vi "AlliGator Reject Source Image ROIs based on Characteristics.vi"(8 "error in (no error)":errorcluster, 10 "ROI Mask Refnum":T1, 11 "Source Image Refnum":T1) -> (0 "error out":errorcluster, 1 "ROI Characteristics String":string)   [LabVIEW 2021, in "AlliGator ROIs.lvlib"]
doc: "Computes ROI characteristics and compare them to the conditions defined by the user in a dialog box.\n\nKeeps only the ROIs that meet those conditions."
uses:
  AlliGator ROIs.lvlib
  <vilib>/vision/Image Controls.llb/IMAQ Image.ctl
  Globals, Variables, Constants/AlliGator Variables List.ctl
  Image/Named ROI Description.ctl
  AlliGator ROI Manager Actions.ctl
  AlliGator Source Image ROI Storage [SGL] v3.vi
  Globals, Variables, Constants/AlliGator Globals, Variables & Constants.lvlib
  Image/Image.lvlib
  Source Image/AlliGator Source Image.lvlib
  Strings/Strings.lvlib
panel:
  # "see the AlliGator License on the block diagram (Ctrl+E or Window:Show Block Diagram)"
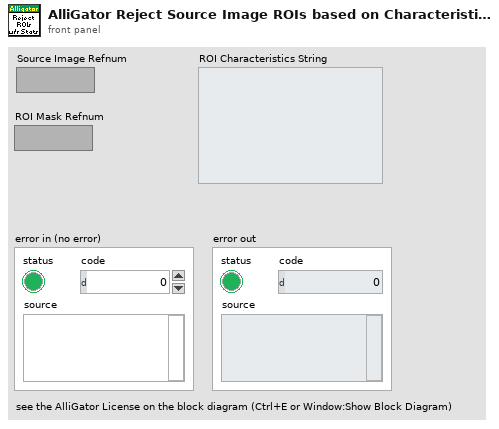
[diagram p1: front panel]
types:
  T1 = typedef "IMAQ Image.ctl" = refnum<image>
  T2 = typedef "Image.lvlib/Named ROI Description.ctl" = cluster{"ROI Descriptor":T3, "ROI Name":string, "Overlay Color":u32}
  T3 = typedef "ROI Descriptor" = cluster{"Global Rectangle":i32[], "Contours":cluster{"ID":enum32{"External", "Internal"}, "Type":u32, "Coordinates":i32[]}[]}
  T4 = typedef "AlliGator Globals, Variables & Constants.lvlib/AlliGator Variables List.ctl" = enum16{"---- GUI ----", "GUI:Initialization Status", "GUI:State Indicators Refnum", "GUI:Original AlliGator Menu Items", "GUI:Current Action Loop State", "GUI:Script in progress", "GUI:Playback", "GUI:Loop Playback", "GUI:Search ROI Used", "GUI:Search ROI", "Decay Graph Max Legend Size", "Intensity Graph Max Legend Size", "Decay Statistics Graph Max Legend Size", "Phasor Graph Max Legend Size", "Phasor Ratio Graph Max Legend Size", "Lifetime Graph Max Legend Size", "---- Files ----", "Files:Export Dataset Frames as Individual Files", "Files:Show Batch Export Help Balloons", "Files:Frames in Dataset", "Files:ptu File Frame Start Indices", "Files:Current Frame in Dataset", "Files:Current Frame Timestamp", "Files:Dataset Loaded", "Files:Dataset Metadata", "Files:Dataset Channel", "Files:Dataset Data Description", "Files:Background Dataset Metadata", "Files:Background Dataset Channel", "Files:Background Dataset Data Description", "Files:Background File Subtraction", "Files:Background File Path", "Files:Background File Pile-up Correction", "Files:Background File Pixel Well Capacity", "Files:Background File Scaling Factor", "Files:Current Dataset Load Settings", "Files:Dataset Path", "Files:ICCD-specific Information", "Files:Macrotime Gate Separation", "------ Python Plugins ------", "Python Plugins:Information", "Python Plugins:Python Session", "Python Plugins:Valid Python Session?", "---- Source Image ----", "Source Image:ROIs", "Source Image:Current ROI", "Source Image:ROI Event Refnum", "X_Source Image Display Range", "X_Source Image Palette Information", "X_Type of Displayed Image", "X_Time Gate Slider", "Source Image:Palette List", "Source Image:Scale", "Source Image:ROI Overlay Color", "Source Image:Overlay to Erase", "Source Image:Is Displayed Image Accumulated", "Source Image:White Light Image Modified", "Source Image:Mask Image Modified", "---- Image Profile Window ----", "Image Profile:Window Event Refnum", "Image Profile:IntensityType", "Image Profile:Intensity Average Type", "Image Profile:Intensity-weighted SDV", "Image Profile:Box Profile Type", "Image Profile:Window Open", "Image Profile:Plotted Fit Parameter", "------ Phasor Graph -------", "Phasor Graph:Show Line", "---- Phasor Plot ---", "Phasor Plot:Parameters Changed", "Phasor Plot:FLI Dataset Modified since last Calculation", "Phasor Harmonics Data", "Selected Phasor Harmonics", "Phasor Harmonic Manager Event Refnum", "Phasor Plot:ROIs", "Phasor Plot:Current ROI", "Phasor Plot:ROI Event Refnum", "Phasor Plot:Image Reference Points", "Phasor Plot:Computed", "Phasor Plot:Palette Information", "Phasor Plot:Palette List", "Phasor Plot:Phasor Ratio Palette Information", "Phasor Plot:Phasor Ratio Palette List", "Phasor Plot:Image Scale", "Phasor Plot:Image Overlay to Erase", "Phasor Plot:Image Elements to Update", "Phasor Plot:Current Calculation Parameters", "Phasor Plot:Current Calibration Options", "Phasor Plot:Reset Cumulated Phasor Plot", "Phasor Plot:Reference 1", "Phasor Plot:Lifetime Reference 1", "Phasor Plot:Reference 1 Frequency", "Phasor Plot:Reference 2", "Phasor Plot:Lifetime Reference 2", "Phasor Plot:Reference 2 Frequency", "---- Decay Analysis ----", "Number of Selected Decays to Fit", "LS Fit Results", "LAR Fit Results", "BS Fit Results", "Last Decay Max - Min", "Best Fit Parameters", "Best Fit Parameter Names", "Actual Size X", "Actual Size Y", "Binning X", "Binning Y", "Actual # Gates", "Dataset Number", "Gates to...", "Gates Skipped", "Gates to keep", "Gate Step", "Gate Separation", "Reversed Gates", "Pile-up Correction", "Pixel Well Capacity", "Background Subtracted", "Background Subtraction Method", "Background Definition Range", "Background File (deprecated)", "Number of Dataset Accumulated", "Array of Accumulated Dataset Paths", "Do Averaged Datasets", "Destination File Path", "Process Plot Target", "Use 1/D as Phasor Frequency", "---- Decay Fit Parameter Map -----", "Decay Fit Parameter Map:Palette Information", "Decay Fit Parameter Map:Palette List", "---- Parameter Map ----", "Parameter Map:Palette Information", "Parameter Map:Palette List", "------- Local Decay Window ---------", "Local Decay Graph Window:Event Refnum", "Local Decay Graph Window:Use normalized IRF for convolution", "----- Miscellaneous ----", "Misc:Skippable Dialog Windows Status"}
  T5 = typedef "AlliGator ROIs.lvlib/AlliGator ROI Manager Actions.ctl" = enum16{"Undefined", "Delete Current ROI", "Delete All Unselected ROIs", "Delete Multiple ROIs", "Delete All ROIs", "Swap ROIs", "Insert ROI", "Update Current ROI Descriptor", "Rename Current ROI", "Store New ROI", "Store Multiple ROIs", "Select Next ROI", "Select Previous ROI", "Find Selected ROI", "Show All ROIs", "Update ROI Manager Window", "Merge All ROIs", "Unmerge ROI", "Set Selected ROI by ID"}
  T6 = typedef "Image.lvlib/Image ROI Statistics.ctl" = cluster{"Area (pixels)":dbl, "% of Image":dbl, "Total Intensity":dbl, "Mean Intensity":dbl, "Median Intensity":dbl, "Mode Intensity":dbl, "Intensity Standard Deviation":dbl, "Min Intensity":dbl, "Max Intensity":dbl, "Mean SNR":dbl, "Median SNR":dbl, "Mode SNR":dbl, "SNR Standard Deviation":dbl, "Max SNR":dbl, "Min SNR":dbl, "# Rejected Pixels (NaN, Inf)":dbl, "# Negative Pixels":dbl, "Long Axis Length":dbl, "Short Axis Length":dbl, "Aspect Ratio":dbl}
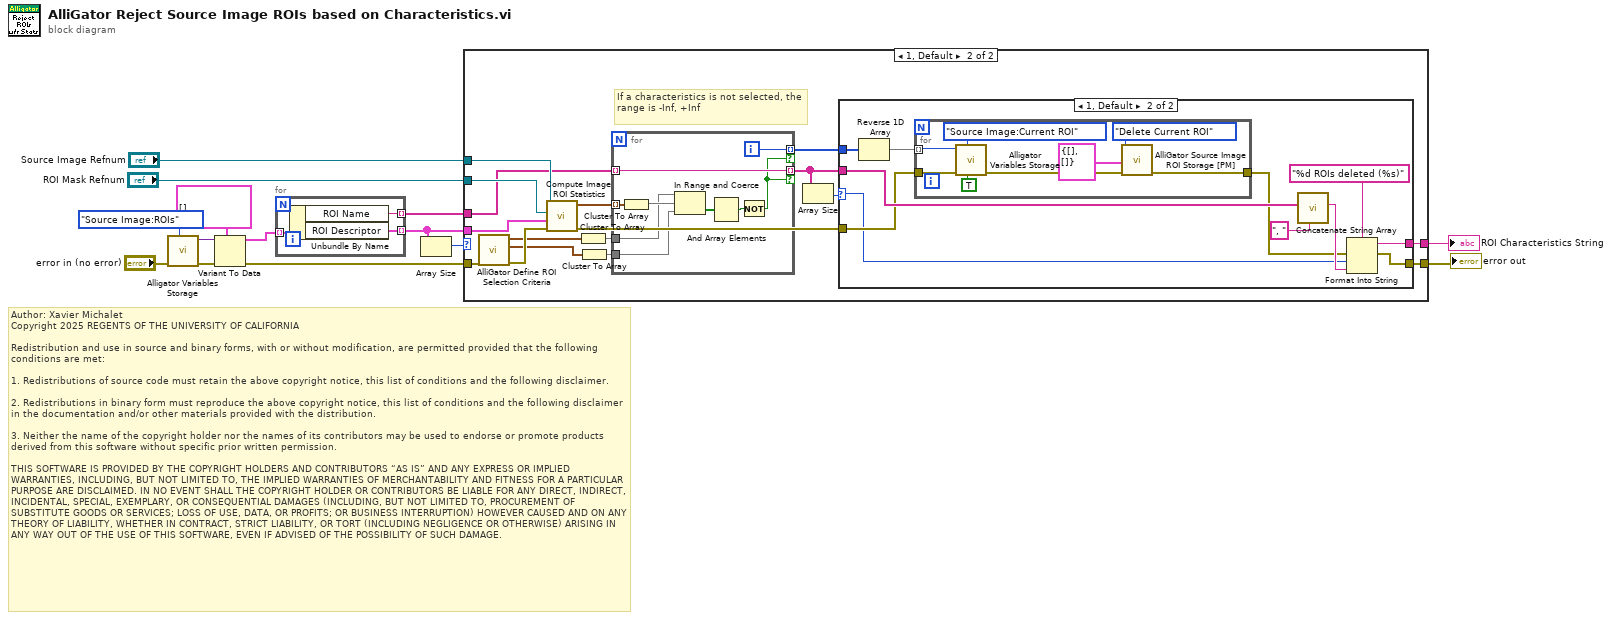
[diagram p0: block diagram]
diagram:
  # "Author: Xavier Michalet\nCopyright 2025 REGENTS OF THE UNIVERSITY OF CALIFORNIA\n\nRedistribution and use in source and binary forms, with or without modification, are permitted provided that the following conditions are met:\n\n1. Redistributions of source code must retain the above copyright notice, this list of conditions and the following disclaimer.\n\n2. Redistributions in binary form must reproduce the above copyright notice, this list of conditions and the following disclaimer in the documentation and/or other materials provided with the distribution.\n\n3. Neither the name of the copyright holder nor the names of its contributors may be used to endorse or promote products derived from this software without specific prior written permission.\n\nTHIS SOFTWARE IS PROVIDED BY THE COPYRIGHT HOLDERS AND CONTRIBUTORS “AS IS” AND ANY EXPRESS OR IMPLIED WARRANTIES, INCLUDING, BUT NOT LIMITED TO, THE IMPLIED WARRANTIES OF MERCHANTABILITY AND FITNESS FOR A PARTICULAR PURPOSE ARE DISCLAIMED. IN NO EVENT SHALL THE COPYRIGHT HOLDER OR CONTRIBUTORS BE LIABLE FOR ANY DIRECT, INDIRECT, INCIDENTAL, SPECIAL, EXEMPLARY, OR CONSEQUENTIAL DAMAGES (INCLUDING, BUT NOT LIMITED TO, PROCUREMENT OF SUBSTITUTE GOODS OR SERVICES; LOSS OF USE, DATA, OR PROFITS; OR BUSINESS INTERRUPTION) HOWEVER CAUSED AND ON ANY THEORY OF LIABILITY, WHETHER IN CONTRACT, STRICT LIABILITY, OR TORT (INCLUDING NEGLIGENCE OR OTHERWISE) ARISING IN ANY WAY OUT OF THE USE OF THIS SOFTWARE, EVEN IF ADVISED OF THE POSSIBILITY OF SUCH DAMAGE."
  n1 = call "Alligator Variables Storage.vi"("AlliGator Variable"=AlliGator_Variables_List."Source Image:ROIs" ("Alligator Variable"), "Error In"="error in (no error)") -> ("Error Out"=w10:errorcluster, "Data out"=w9:variant)  [unwired: 7 in, 1 out]
  n2 = Variant To Data(error in=w10, type=T2[] [] ("Stored ROIs in"), Variant=w9) -> (data=w12:T2[], error out=w5:errorcluster)
  n3 = for {
    tunnel: w12 -> [w17] mode=indexing
    tunnel: [w16] -> w3 mode=indexing
    tunnel: [w15] -> w1 mode=indexing
    n4 = Unbundle By Name(w17) -> ("ROI Name"=w15:string, "ROI Descriptor"=w16:T3)
  }
  n5 = Array Size(array=w3) -> (size(s)=w2:i32)
  n6 = case shown="1, Default" w2 {
    tunnel: "ROI Mask Refnum" -> [_ w35]
    tunnel: "Source Image Refnum" -> [_ w34]
    tunnel: [w18 w32] -> w7
    tunnel: [_ w31] -> w6
    tunnel: w5 -> [w18 w30]
    tunnel: w3 -> [_ w28]
    tunnel: w1 -> [_ w24]
    frame 0 {
      # "no ROIs"
    }
    frame 1, Default {
      # "If a characteristics is not selected, the range is -Inf, +Inf"
      n7 = call "AlliGator Define ROI Selection Criteria.vi"("Error In"=w30) -> ("Error Out"=w29:errorcluster, "ROI Characteristics Min out"=w19:T6, "ROI Characteristics Max out"=w27:T6)  [unwired: 7 in, 1 out]
      n8 = call "Compute Image ROI Statistics.vi"("error in (no error)"=w29, "ROIs"=w28, "ROI Mask Refnum"=w35, "Image Refnum"=w34) -> ("error out"=w23:errorcluster, "ROI Characteristics"=w33:T6[])  [unwired: 5 in, 1 out]
      n9 = Cluster To Array(cluster=w27) -> (array=w26:dbl[])
      n10 = Cluster To Array(cluster=w19) -> (array=w25:dbl[])
      n11 = for {
        tunnel: w33 -> [w64] mode=indexing
        tunnel: w26 -> [w62]
        tunnel: w25 -> [w57]
        tunnel: w24 -> [w61] mode=indexing
        tunnel: [w61] -> w21 mode=indexing if=w59
        tunnel: [w60] -> w22 mode=indexing if=w59
        i -> [w60]
        n12 = Cluster To Array(cluster=w64) -> (array=w63:dbl[])
        n13 = In Range and Coerce(upper limit=w62, x=w63, lower limit=w57) -> (In Range?=w56:bool[])  [unwired: 1 out]
        n14 = And Array Elements(Boolean array=w56) -> (logical AND=w58:bool)
        n15 = Not(x=w58) -> (.not. x?=w59:bool)
      }
      n16 = Array Size(array=w21) -> (size(s)=w20:i32)
      n17 = case shown="1, Default" w20 {
        selector: w20 -> [_ w37]
        tunnel: [w36 w47] -> w32
        tunnel: [_ w46] -> w31
        tunnel: w21 -> [_ w40]
        tunnel: w23 -> [w36 w39]
        tunnel: w22 -> [_ w42]
        frame 0 {
        }
        frame 1, Default {
          n18 = Reverse 1D Array(array=w42) -> (reversed array=w41:i32[])
          n19 = for {
            tunnel: w41 -> [w54] mode=indexing
            tunnel: w39 -> [w49]
            tunnel: [w48] -> w38
            n20 = call "Alligator Variables Storage.vi"("Get(F)/Set"=TRUE, "AlliGator Variable"=AlliGator_Variables_List."Source Image:Current ROI" ("Alligator Variable"), "Error In"=w49, "Data in"=w54) -> ("Error Out"=w52:errorcluster)  [unwired: 5 in, 2 out]
            n21 = call-poly "AlliGator Source Image ROI Storage [PM].vi"("Error In"=w52, "Current ROI Descriptor"=T3 {"Global Rectangle"=[], "Contours"=[]}, "Action"=AlliGator_ROI_Manager_Actions."Delete Current ROI") -> ("Error Out"=w48:errorcluster)  [unwired: 2 in, 6 out]
          }
          n22 = call "Concatenate String Array.vi"("Separator (TAB)"=", ", "String Array"=w40) -> ("Formatted String"=w43:string)  [unwired: 9 in]
          n23 = Format Into String(format string="%d ROIs deleted (%s)", error in=w38, w37, w43) -> (resulting string=w46:string, error out=w47:errorcluster)  [unwired: 1 in]
        }
      }
    }
  }
  "ROI Characteristics String" <- w6
  "error out" <- w7
